vi "Read Names.vi"(11 "Effect Interface in":refnum<class "Effect Interface.lvclass">) -> (0 "Value2 Name":string, 1 "Value1 Name":string, 2 "Effect Name":string, 3 "Effect Interface out":refnum<class "Effect Interface.lvclass">)   [LabVIEW 2019, in "Effect Interface.lvlib" / "Effect Interface.lvclass"]
uses:
  Effect Interface.lvclass
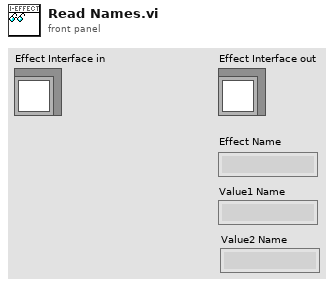
[diagram p1: front panel]
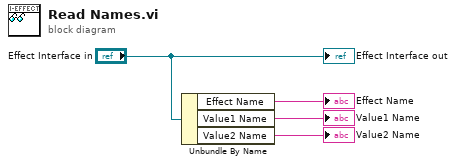
[diagram p0: block diagram]
diagram:
  n1 = Unbundle By Name("Effect Interface in") -> ("Effect Name"=→"Effect Name":string, "Value1 Name"=→"Value1 Name":string, "Value2 Name"=→"Value2 Name":string)
  "Effect Interface out" <- "Effect Interface in"
